vi "Sub Img RGBA to RGB.vi"(10 "Default Color":u32(colorbox), 11 "RGBA Array":u8[](array[numeric])) -> (3 "RGB Array":cluster{"R":u8, "G":u8, "B":u8}[](array[cluster]))   [LabVIEW 2018, in "Image Process.lvclass"]
uses:
  Image Process.lvclass
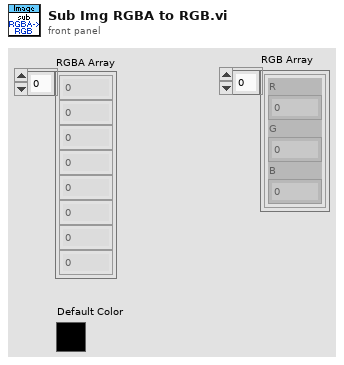
[diagram p1: front panel]
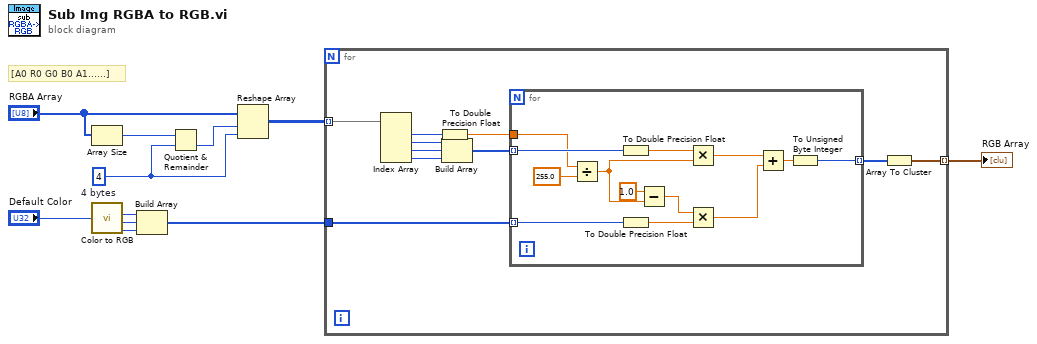
[diagram p0: block diagram]
diagram:
  w8 = 4  # 4 bytes
  # "[A0 R0 G0 B0 A1......]"
  n1 = Array Size(array="RGBA Array") -> (size(s)=w11:i32)
  n2 = call <vilib>:"Color to RGB.vi"("Color"="Default Color") -> ("R"=w5:u8, "G"=w4:u8, "B"=w3:u8)  [unwired: 1 out]
  n3 = Build Array(w5, w4, w3) -> (w1:u8[])
  n4 = Quotient & Remainder(x=w11, y=w8) -> (floor(x/y)=w10:i32)  [unwired: 1 out]
  n5 = Reshape Array("RGBA Array", w10, w8) -> (w7:u8[][])
  n6 = for {
    tunnel: w7 -> [w20] mode=indexing
    tunnel: w1 -> [w21]
    tunnel: [w15] -> w2 mode=indexing
    n7 = Index Array(array=w20) -> (element #1=w12:u8, element #2=w19:u8, element #3=w18:u8, element #4=w17:u8)  [unwired: 4 in]
    n8 = To Double Precision Float(number=w12) -> (double precision float=w13:dbl)
    n9 = Build Array(w19, w18, w17) -> (w16:u8[])
    n10 = for {
      tunnel: w21 -> [w31] mode=indexing
      tunnel: w16 -> [w34] mode=indexing
      tunnel: [w22] -> w14 mode=indexing
      tunnel: w13 -> [w28]
      n11 = Divide(x=w28, y=255.0) -> (x/y=w24:dbl)
      n12 = To Double Precision Float(number=w34) -> (double precision float=w29:dbl)
      n13 = To Double Precision Float(number=w31) -> (double precision float=w26:dbl)
      n14 = Subtract(x=1.0, y=w24) -> (x-y=w32:dbl)
      n15 = Multiply(x=w29, y=w24) -> (x*y=w33:dbl)
      n16 = Multiply(x=w32, y=w26) -> (x*y=w23:dbl)
      n17 = Add(x=w33, y=w23) -> (x+y=w30:dbl)
      n18 = To Unsigned Byte Integer(number=w30) -> (unsigned 8bit integer=w22:u8)
    }
    n19 = Array To Cluster(array=w14) -> (cluster=w15:cluster{"[0]":u8, "[1]":u8, "[2]":u8})
  }
  "RGB Array" <- w2
